vi "pressure_time_plotting.vi"(0 "file path (use dialog)":path, 1 "Valve Open Time / s":dbl, 2 "Valve Close Time / s":dbl, 3 "End scan time / s":dbl, 11 "error in (no error)":errorcluster, 12 "Set Flow / mbar ls-1":dbl, 14 "Target Recording Frequency / Hz":i32) -> (15 "error out":errorcluster)   [LabVIEW 2019]
uses:
  <vilib>/Utility/file.llb/Write Delimited Spreadsheet (DBL).vi
panel:
  out "Loop Execution Time / ms":u32
  out "Pressure Time Dependance":cluster{dbl[], dbl[]}(graph)
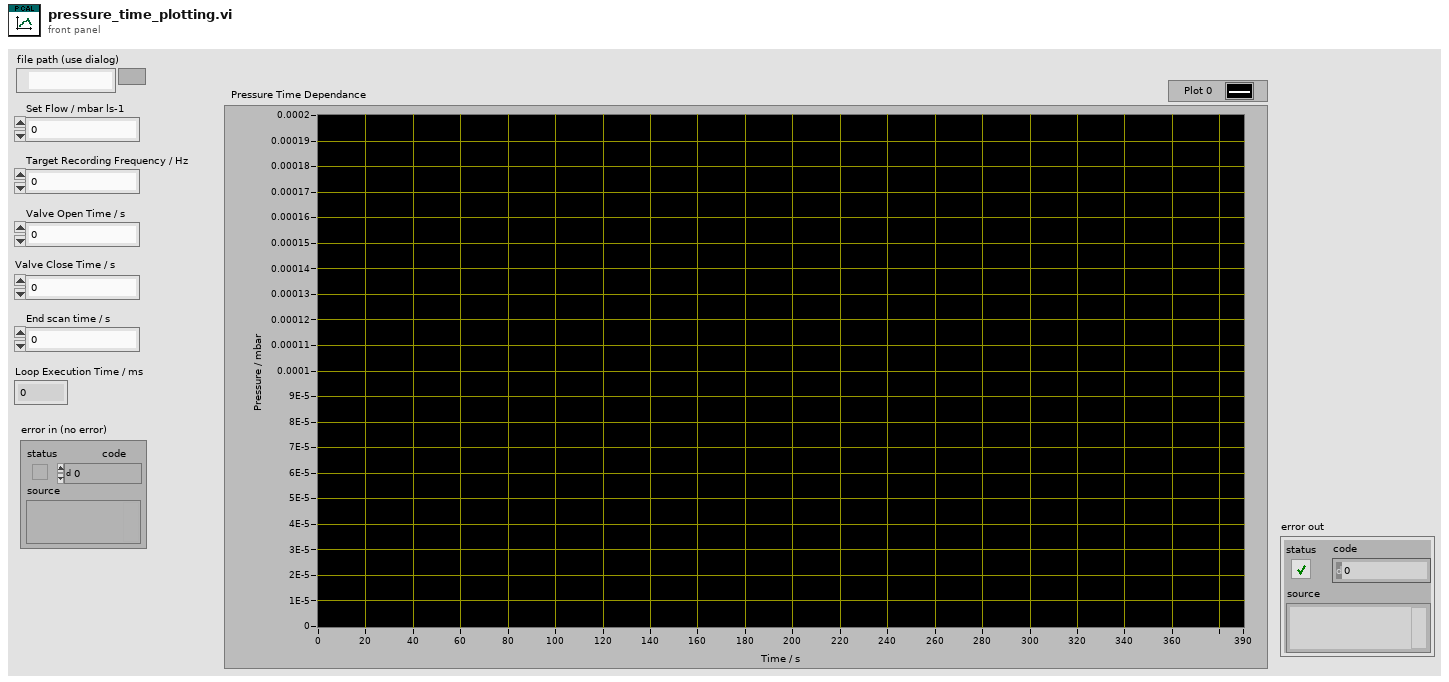
[diagram p1: front panel]
types:
  T1 = enum16{"open", "replace", "create", "open or create", "replace or create", "replace or create with confirmation"}
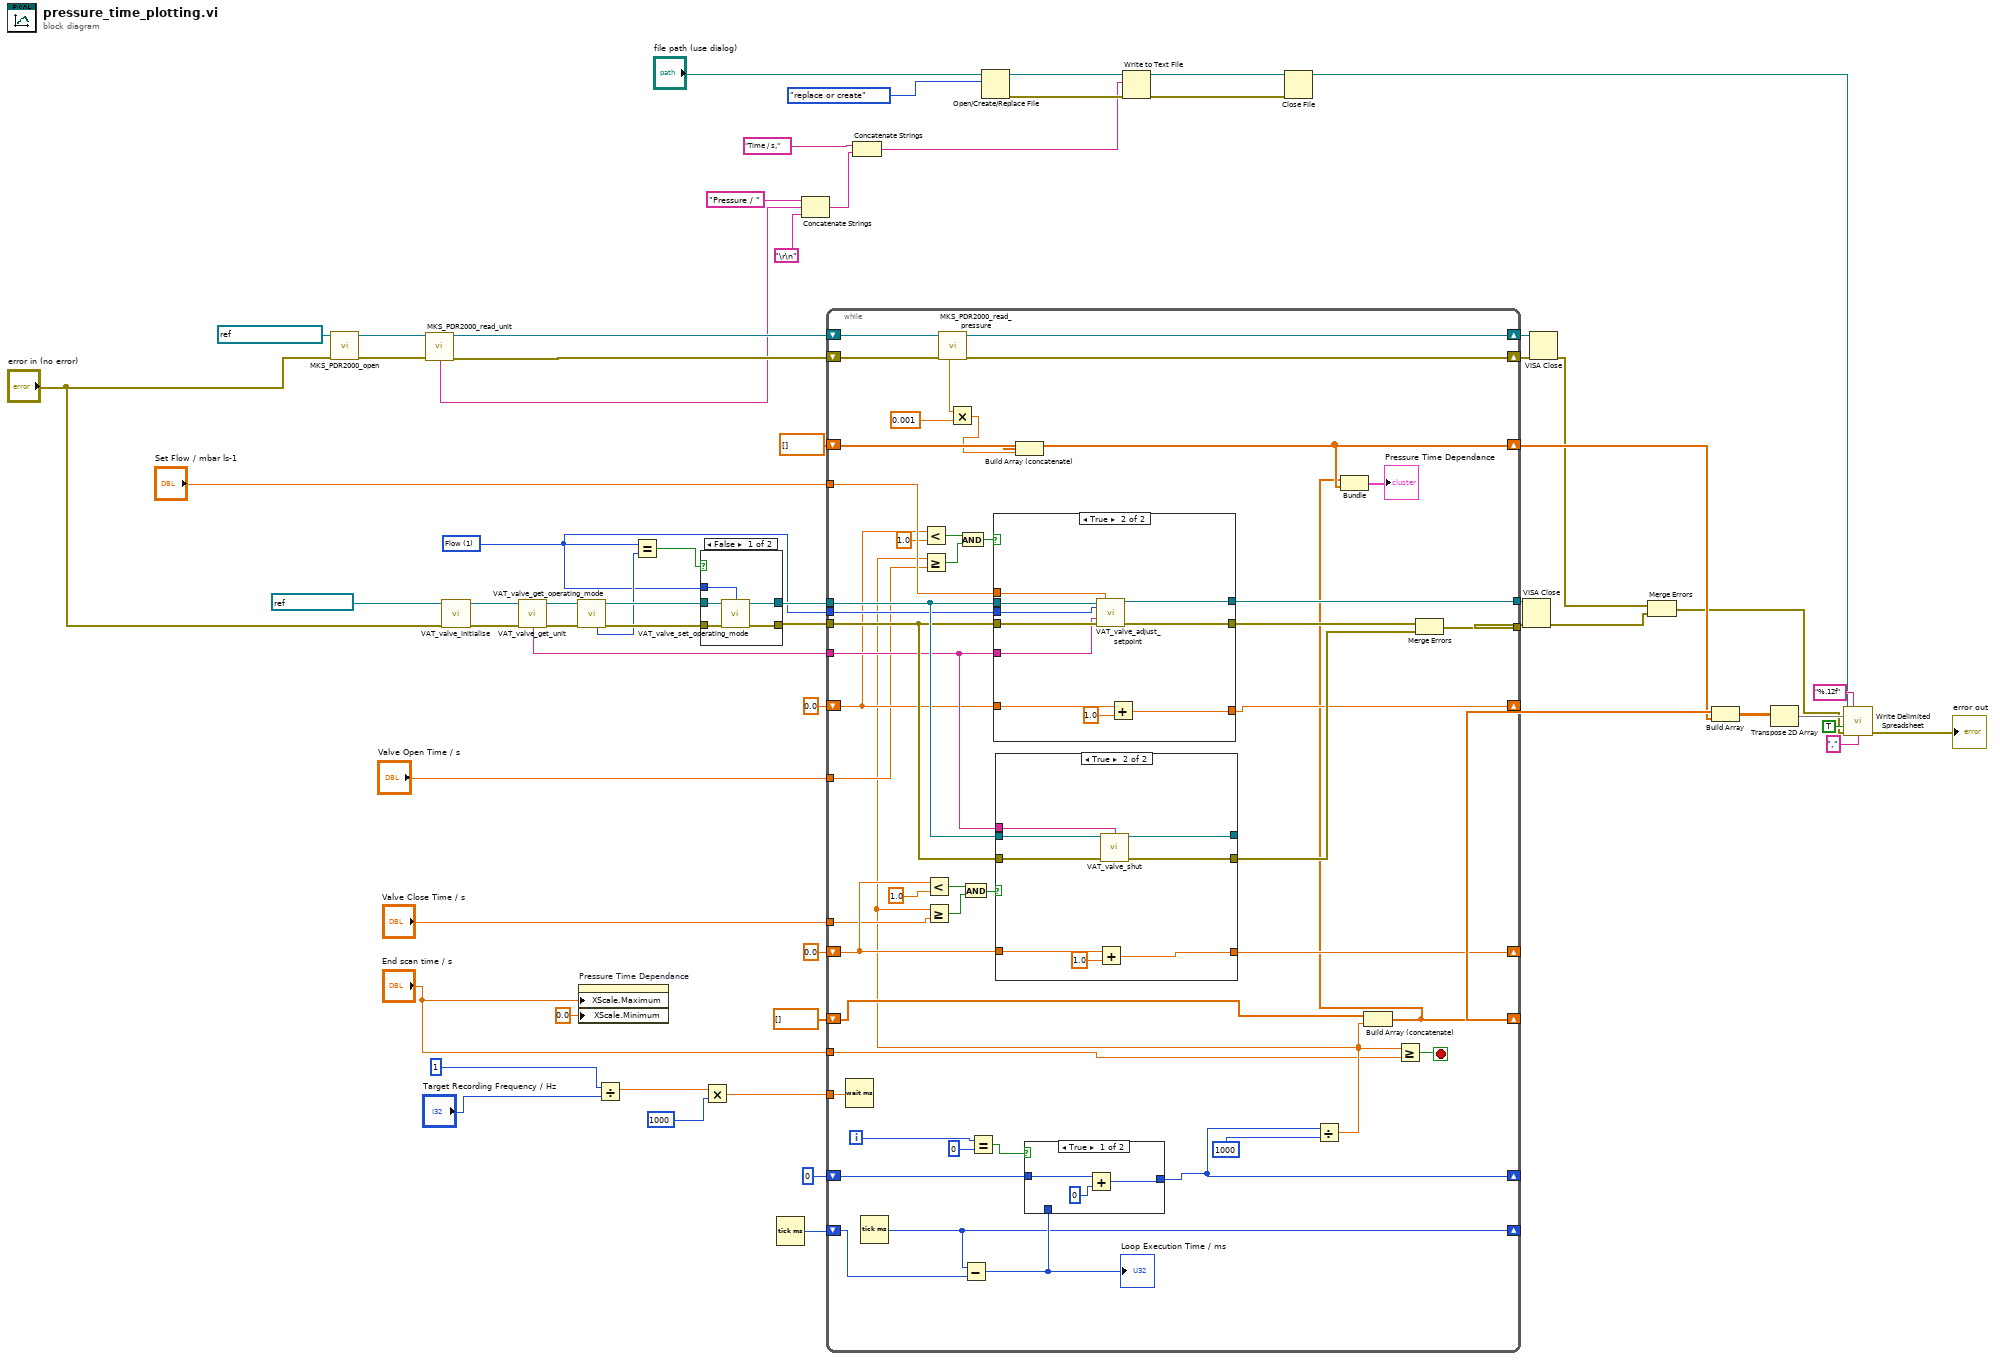
[diagram p0: block diagram]
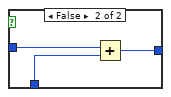
[diagram p3: hidden frame]
diagram:
  w38 = u16 1 items=["Pressure", "Flow", "Stop"] ("Operating Mode")
  n1 = call "MKS_PDR2000_open.vi"("error in (no error)"="error in (no error)", "PDR2000 COM port"=refnum<visa-resource-name> "PDR_2000") -> ("error out"=w61:errorcluster, "PDR2000 COM port out"=w62:refnum<visa-resource-name>)  [unwired: 8 in]
  n2 = call "MKS_PDR2000_read_unit.vi"("PDR2000 COM port"=w62, "error in (no error)"=w61) -> ("PDR2000 COM port out"=w41:refnum<visa-resource-name>, "Unit"=w6:string, "error out"=w40:errorcluster)  [unwired: 11 in]
  n3 = call "VAT_valve_initialise.vi"("VAT Valve COM port"=refnum<visa-resource-name> "VAT_valve", "error in (no error)"="error in (no error)") -> ("VAT Valve COM port out"=w53:refnum<visa-resource-name>, "error out"=w52:errorcluster)  [unwired: 6 in, 6 out]
  n4 = call "VAT_valve_get_unit.vi"("VAT Valve COM port"=w53, "error in (no error)"=w52) -> ("VAT Valve COM port out"=w51:refnum<visa-resource-name>, "Unit"=w37:string, "error out"=w50:errorcluster)  [unwired: 11 in]
  n5 = call "VAT_valve_get_operating_mode.vi"("VAT Valve COM port"=w51, "error in (no error)"=w50) -> ("VAT Valve COM port out"=w49:refnum<visa-resource-name>, "Operating Mode"=w46:u16, "error out"=w48:errorcluster)  [unwired: 10 in, 1 out]
  n6 = property on="Pressure Time Dependance" class="XYGraph (strict)"("XScale.Maximum"="End scan time / s", "XScale.Minimum"=0.0 ("X Scale.Range:Minimum")) -> ()  [unwired: 2 in, 2 out]
  n7 = Divide(x=1, y="Target Recording Frequency / Hz") -> (x/y=w26:dbl)
  n8 = Equal?(x=w38, y=w46) -> (x = y?=w47:bool)
  n9 = case shown="False" w47 {
    tunnel: w49 -> [w68 w70]
    tunnel: w48 -> [w67 w69]
    tunnel: [w66 w70] -> w45
    tunnel: [w65 w69] -> w44
    tunnel: w38 -> [w64 _]
    frame False {
      n10 = call "VAT_valve_set_operating_mode.vi"("VAT Valve COM port"=w68, "Operating Mode"=w64, "error in (no error)"=w67) -> ("VAT Valve COM port out"=w66:refnum<visa-resource-name>, "error out"=w65:errorcluster)  [unwired: 11 in]
    }
    frame True {
    }
  }
  n11 = Multiply(x=w26, y=1000 ("x")) -> (x*y=w57:dbl)
  n12 = Tick Count (ms)() -> (millisecond timer value=w22:u32)
  n13 = Concatenate Strings("Pressure / " ("string"), w6, "\r\n") -> (w13:string)
  n14 = while {
    shift-right: [w116] -> w60
    shift-left: w41 -> [w118]
    shift-right: [w115] -> w59
    shift-left: w40 -> [w117]
    tunnel: w57 -> [w104]
    shift-right: [w86] -> w31
    shift-left: dbl[] [] -> [w114]
    tunnel: w45 -> [w113]
    tunnel: w44 -> [w112]
    tunnel: [w111] -> w43
    tunnel: [w108] -> w42
    tunnel: "Set Flow / mbar ls-1" -> [w107]
    tunnel: w38 -> [w106]
    tunnel: w37 -> [w105]
    shift-right: [w103] -> _
    shift-left: 0.0 -> [w100]
    tunnel: "Valve Open Time / s" -> [w97]
    shift-right: [w96] -> _
    shift-left: 0.0 -> [w91]
    tunnel: "Valve Close Time / s" -> [w90]
    tunnel: "End scan time / s" -> [w74]
    shift-right: [w84] -> w32
    shift-left: dbl[] [] -> [w85]
    shift-right: [w77] -> _
    shift-left: u32 0 ("millisecond timer value") -> [w81]
    shift-right: [w78] -> _
    shift-left: w22 -> [w80]
    i -> [w73]
    stop <- w82 stop-if-true
    n15 = Wait (ms)(milliseconds to wait=w104) -> ()  [unwired: 1 out]
    n16 = Tick Count (ms)() -> (millisecond timer value=w78:u32)
    n17 = Less?(x=w100, y=1.0) -> (x < y?=w101:bool)
    n18 = Less?(x=w91, y=1.0) -> (x < y?=w95:bool)
    n19 = call "MKS_PDR2000_read_pressure.vi"("error in (no error)"=w117, "PDR2000 COM port"=w118) -> ("error out"=w115:errorcluster, "PDR2000 COM port out"=w116:refnum<visa-resource-name>, "Channel 1 Pressure"=w88:dbl)  [unwired: 6 in, 1 out]
    n20 = Multiply(x=w88, y=0.001) -> (x*y=w87:dbl)
    n21 = Subtract(x=w78, y=w80) -> (x-y=w79:u32)
    "Loop Execution Time / ms" <- w79
    n22 = Equal?(x=w73, y=0) -> (x = y?=w71:bool)
    n23 = Build Array (concatenate)(w114, w87) -> (w86:dbl[])
    n24 = case shown="True" w71 {
      tunnel: w81 -> [w121 w124]
      tunnel: w79 -> [_ w123]
      tunnel: [w120 w122] -> w77
      frame True {
        n25 = Add(x=w121, y=0) -> (x+y=w120:u32)
      }
      frame False {
        n26 = Add(x=w124, y=w123) -> (x+y=w122:u32)
      }
    }
    n27 = Divide(x=w77, y=u32 1000) -> (x/y=w75:dbl)
    n28 = Greater Or Equal?(x=w75, y=w97) -> (x >= y?=w98:bool)
    n29 = Greater Or Equal?(x=w75, y=w90) -> (x >= y?=w94:bool)
    n30 = And(x=w101, y=w98) -> (x .and. y?=w102:bool)
    n31 = And(x=w95, y=w94) -> (x .and. y?=w93:bool)
    n32 = case shown="True" w102 {
      tunnel: w113 -> [w138 w148]
      tunnel: w112 -> [w137 w147]
      tunnel: [w138 w146] -> w111
      tunnel: [w137 w145] -> w110
      tunnel: w107 -> [_ w144]
      tunnel: w106 -> [_ w143]
      tunnel: w105 -> [_ w142]
      tunnel: w100 -> [w136 w141]
      tunnel: [w136 w140] -> w103
      frame False {
      }
      frame True {
        n33 = call "VAT_valve_adjust_setpoint.vi"("VAT Valve COM port"=w148, "Flow"=w144, "Operating Mode"=w143, "Unit"=w142, "error in (no error)"=w147) -> ("VAT Valve COM port out"=w146:refnum<visa-resource-name>, "error out"=w145:errorcluster)  [unwired: 9 in]
        n34 = Add(x=w141, y=1.0) -> (x+y=w140:dbl)
      }
    }
    n35 = case shown="True" w93 {
      tunnel: w113 -> [w127 w135]
      tunnel: w112 -> [w126 w134]
      tunnel: [w126 w133] -> w109
      tunnel: w105 -> [_ w132]
      tunnel: [w127 w131] -> _
      tunnel: [w125 w130] -> w96
      tunnel: w91 -> [w125 w129]
      frame False {
      }
      frame True {
        n36 = Add(x=w129, y=1.0) -> (x+y=w130:dbl)
        n37 = call "VAT_valve_shut.vi"("VAT Valve COM port"=w135, "Unit"=w132, "error in (no error)"=w134) -> ("VAT Valve COM port out"=w131:refnum<visa-resource-name>, "error out"=w133:errorcluster)  [unwired: 10 in, 1 out]
      }
    }
    n38 = Build Array (concatenate)(w85, w75) -> (w84:dbl[])
    n39 = Bundle(w84, w86) -> (→"Pressure Time Dependance":cluster{dbl[], dbl[]})  [unwired: 1 in]
    n40 = Greater Or Equal?(x=w75, y=w74) -> (x >= y?=w82:bool)
    n41 = Merge Errors(w110, w109) -> (w108:errorcluster)
  }
  n42 = Concatenate Strings("Time / s,", w13) -> (w12:string)
  n43 = Open/Create/Replace File(file path (use dialog)="file path (use dialog)", operation (0:open)=T1."replace or create") -> (refnum out=w21:refnum<file>, error out=w20:errorcluster)  [unwired: 4 in, 1 out]
  n44 = Write to Text File(file (use dialog)=w21, text=w12, error in=w20) -> (refnum out=w19:refnum<file>, error out=w18:errorcluster)  [unwired: 1 in, 1 out]
  n45 = Close File(refnum=w19, error in=w18) -> (path=w14:path)  [unwired: 1 out]
  n46 = VISA Close(VISA resource name=w43, error in (no error)=w42) -> (error out=w8:errorcluster)
  n47 = VISA Close(VISA resource name=w60, error in (no error)=w59) -> (error out=w9:errorcluster)
  n48 = Merge Errors(w9, w8) -> (w7:errorcluster)
  n49 = Build Array(w32, w31) -> (w30:dbl[][])
  n50 = Transpose 2D Array(2D array=w30) -> (transposed array=w29:dbl[][])
  n51 = call-poly <vilib>:"Write Delimited Spreadsheet.vi"("file path (dialog if empty)"=w14, "format (%.3f)"="%.12f", "2D data"=w29, "append to file? (new file:F)"=TRUE, "error in (no error)"=w7, "delimiter (\\t)"="," ("delimiter (\\t)")) -> ("error out"=→"error out":errorcluster)  [unwired: 8 in, 1 out]
